vi "Realsense Cam Update Stream Profiles.vi"(8 "error in (no error)":errorcluster, 11 "Realsense Cam in":refnum<class "Realsense Cam.lvclass">) -> (0 "error out":errorcluster, 3 "Realsense Cam out":refnum<class "Realsense Cam.lvclass">)   [LabVIEW 2018, in "Realsense Cam.lvclass"]
uses:
  Realsense Cam.lvclass
  Realsense Cam.lvclass/Realsense Cam.ctl
  realsense_wrapper_api/libRealSense3.lvlib
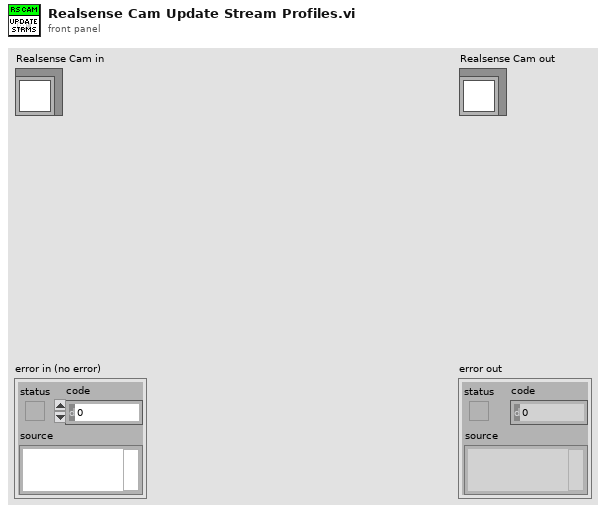
[diagram p1: front panel]
types:
  T1 = cluster{"ID":i32, "Profile":u64, "fps":i32, "RS Stream":u16, "RS Format":u16, "index":u16, "width":u16, "height":u16, "ppx":sgl, "ppy":sgl, "fx":sgl, "fy":sgl, "model":u32}
  T2 = cluster{"width":i32, "height":i32, "fps":i32, "Profile":u64, "ppx":sgl, "ppy":sgl, "fx":sgl, "fy":sgl, "model":u32}[]
  T3 = typedef "Realsense Cam.lvclass/Stream STYP.ctl" = cluster{"Strings":string[], "Intrinsics":cluster{"width":i32, "height":i32, "fps":i32, "Profile":u64, "ppx":sgl, "ppy":sgl, "fx":sgl, "fy":sgl, "model":u32}[], "Current Data":T4}
  T4 = typedef "Realsense Cam.lvclass/Stream Frame Data STYP.ctl" = cluster{"Depths":sgl[][], "Bytes":u8[], "16-Bit IR":u16[], "Height":i32, "Width":i32}
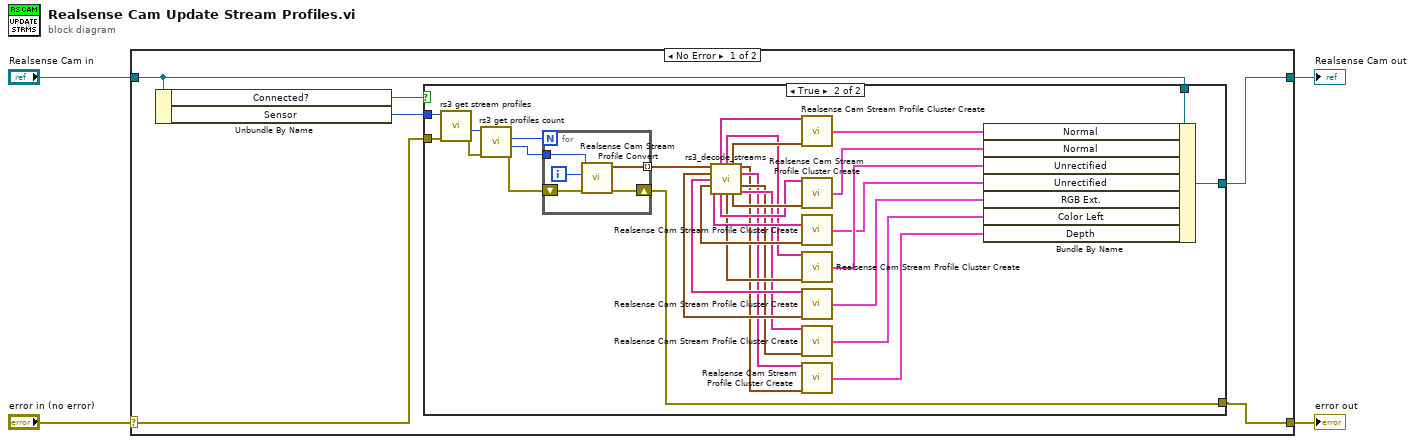
[diagram p0: block diagram]
diagram:
  n1 = case shown="No Error" "error in (no error)" {
    selector: "error in (no error)" -> [w6 w51]
    tunnel: [w5 w51] -> w3
    tunnel: [w8 w50] -> w1
    tunnel: "Realsense Cam in" -> [w7 w50]
    frame No Error {
      n2 = Unbundle By Name(w7) -> ("Connected?"=w10:bool, "Sensor"=w9:u64)
      n3 = case shown="True" w10 {
        tunnel: w9 -> [_ w44]
        tunnel: w6 -> [w11 w43]
        tunnel: w7 -> [w12 w22]
        tunnel: [w12 w14] -> w8
        tunnel: [w11 w13] -> w5
        frame False {
        }
        frame True {
          n4 = call "rs3 get stream profiles.vi"("error in (no error)"=w43, "Sensor in"=w44) -> ("error out"=w41:errorcluster, "Stream profile list"=w42:u64)  [unwired: 6 in, 2 out]
          n5 = call "rs3 get profiles count.vi"("error in"=w41, "Profiles_list"=w42) -> ("error out"=w38:errorcluster, "Profiles_list_out"=w39:u64, "Profiles count"=w40:i32)  [unwired: 6 in, 1 out]
          n6 = for {
            N: w40 -> [_]
            tunnel: w39 -> [w49]
            shift-right: [w46] -> w13
            shift-left: w38 -> [w47]
            tunnel: [w45] -> w37 mode=indexing
            i -> [w48]
            n7 = call "Realsense Cam Stream Profile Convert.vi"("error in (no error)"=w47, "Numeric"=w48, "Profiles_list_out"=w49) -> ("error out"=w46:errorcluster, "output cluster"=w45:T1)  [unwired: 7 in]
          }
          n8 = call "rs3_decode_streams.vi"("Stream profile array"=w37) -> ("IR Left Array"=w35:string[], "Unrectified R IR"=w30:string[], "IR left"=w36:T2, "Depth Stream"=w23:T2, 5:"RGB ext."=w27:T2, "Depth Stream strings"=w24:string[], 7:"RGB ext."=w28:string[], 9:"Unrectified L IR"=w32:T2, "Color Left"=w25:T2, 11:"Unrectified L IR"=w31:string[], "IR Right Array"=w33:string[], "Unrectified R  IR"=w29:T2, "IR Right"=w34:T2, "Color Left Array"=w26:string[])  [unwired: 1 in]
          n9 = call "Realsense Cam Stream Profile Cluster Create.vi"("Strings"=w35, "Intrinsics"=w36) -> ("Stream"=w21:T3)  [unwired: 13 in]
          n10 = call "Realsense Cam Stream Profile Cluster Create.vi"("Strings"=w33, "Intrinsics"=w34) -> ("Stream"=w20:T3)  [unwired: 13 in]
          n11 = call "Realsense Cam Stream Profile Cluster Create.vi"("Strings"=w31, "Intrinsics"=w32) -> ("Stream"=w18:T3)  [unwired: 13 in]
          n12 = call "Realsense Cam Stream Profile Cluster Create.vi"("Strings"=w30, "Intrinsics"=w29) -> ("Stream"=w19:T3)  [unwired: 13 in]
          n13 = call "Realsense Cam Stream Profile Cluster Create.vi"("Strings"=w28, "Intrinsics"=w27) -> ("Stream"=w17:T3)  [unwired: 13 in]
          n14 = call "Realsense Cam Stream Profile Cluster Create.vi"("Strings"=w26, "Intrinsics"=w25) -> ("Stream"=w16:T3)  [unwired: 13 in]
          n15 = call "Realsense Cam Stream Profile Cluster Create.vi"("Strings"=w24, "Intrinsics"=w23) -> ("Stream"=w15:T3)  [unwired: 13 in]
          n16 = Bundle By Name(cluster=w22, "Normal"=w21, "Normal"=w20, "Unrectified"=w19, "Unrectified"=w18, "RGB Ext."=w17, "Color Left"=w16, "Depth"=w15) -> (w14:refnum<class "Realsense Cam.lvclass">)
        }
      }
    }
    frame Error {
    }
  }
  "error out" <- w3
  "Realsense Cam out" <- w1
